vi "质控报警信息存储 (子VI).vi"   [LabVIEW 2016, in "质控单元.lvlib"]
uses:
  <vilib>/ptbypt/NI_PtbyPt.lvlib
types:
  T1 = cluster{"时间标识":timestamp, "设备":string, "日志信息":string, "流程参数":string}
  T2 = cluster{"时间标识":timestamp, "设备":string, "日志信息":string}
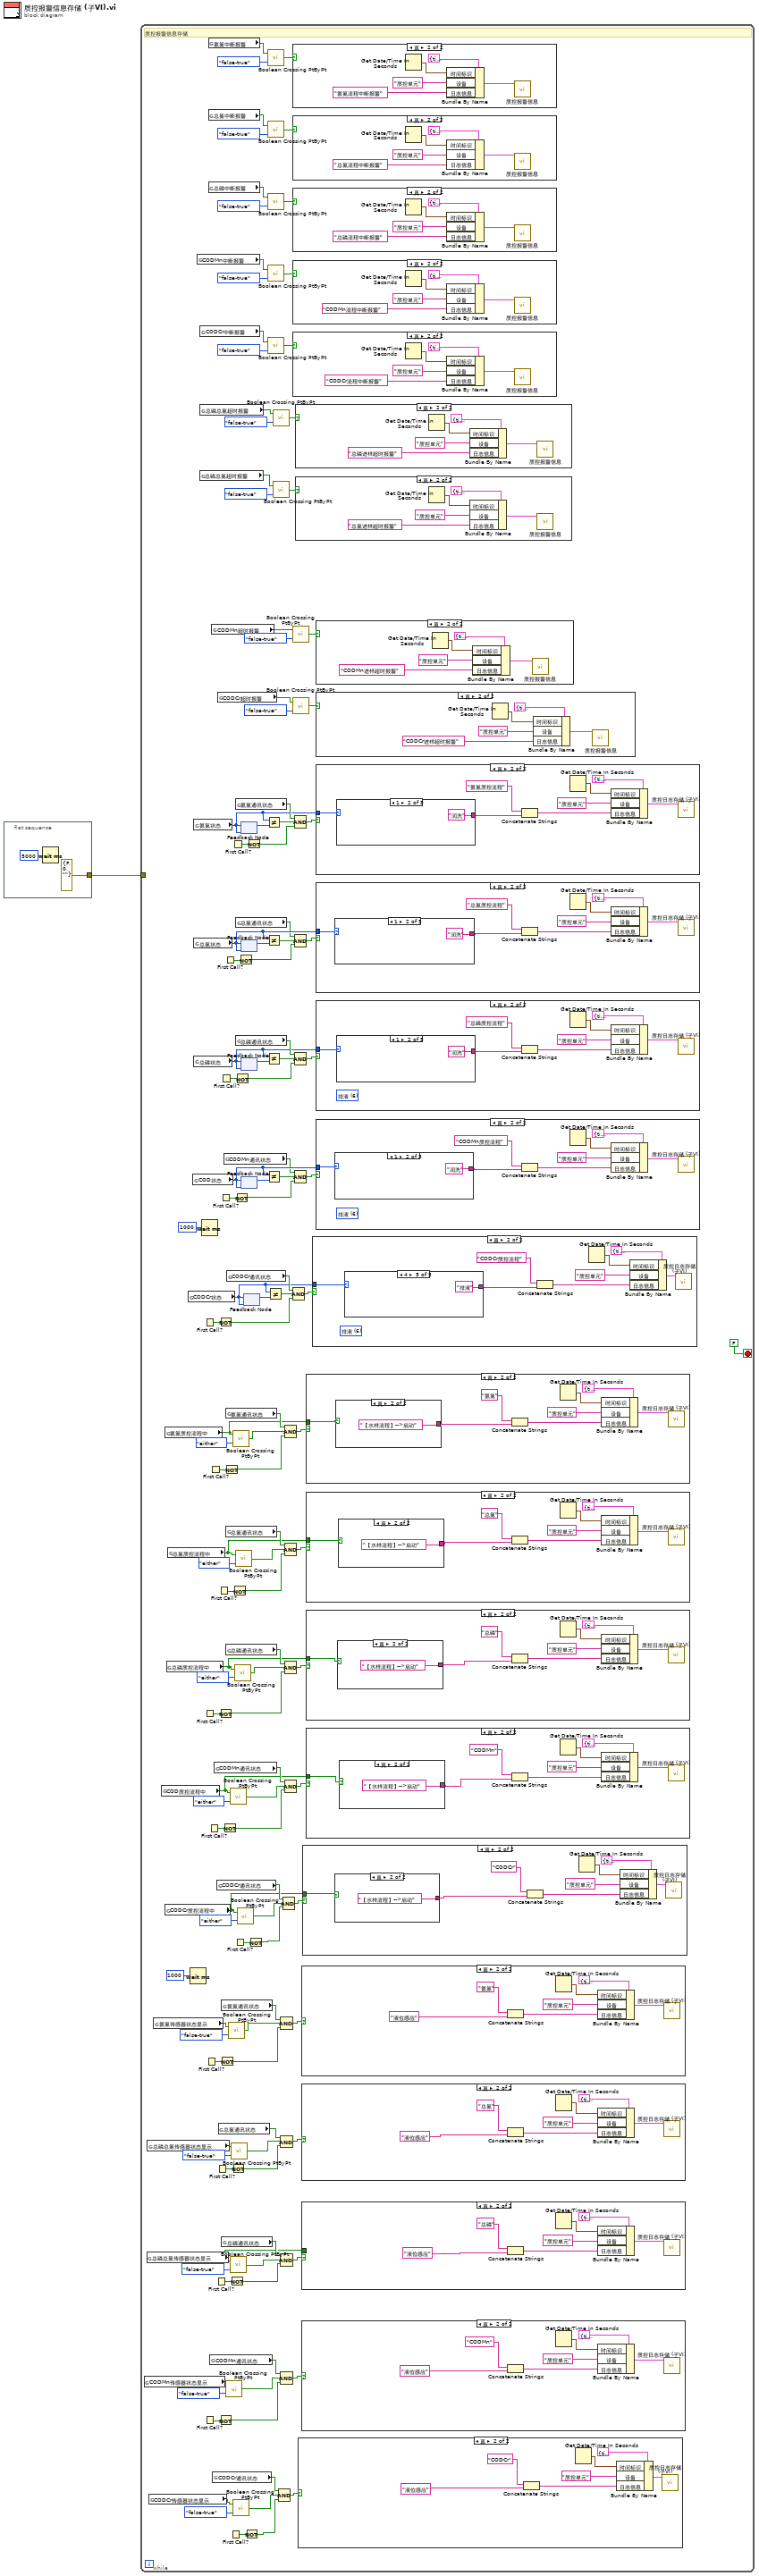
[diagram p0: block diagram]
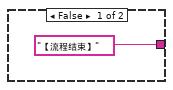
[diagram p8: hidden frame]
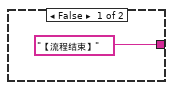
[diagram p10: hidden frame]
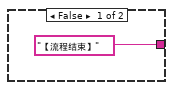
[diagram p12: hidden frame]
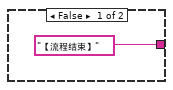
[diagram p14: hidden frame]
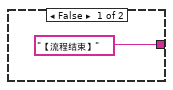
[diagram p16: hidden frame]
diagram:
  n1 = flat-sequence {
    tunnel: [errorcluster {"status"=FALSE, "code"=0, "source"=""} ("错误常量")] -> w1
    frame #0 {
      n2 = Wait (ms)(milliseconds to wait=u32 5000 ("等待时间（毫秒）")) -> ()  [unwired: 1 out]
    }
  }
  n3 = while {
    tunnel: w1 -> [_]
    stop <- FALSE stop-if-true
    # "质控报警信息存储"
    n4 = global read "质控中断报警全局.vi" "CODMn传感器状态显示"() -> (w5:bool)
    n5 = global read "质控中断报警全局.vi" "总磷总氮传感器状态显示"() -> (w6:bool)
    n6 = global read "质控中断报警全局.vi" "总磷总氮传感器状态显示"() -> (w7:bool)
    n7 = global read "质控中断报警全局.vi" "CODCr传感器状态显示"() -> (w4:bool)
    n8 = global read "质控中断报警全局.vi" "氨氮传感器状态显示"() -> (w8:bool)
    n9 = global read "质控测完标志全局 1.vi" "COD质控流程中"() -> (w42:bool)
    n10 = global read "质控测完标志全局 1.vi" "氨氮质控流程中"() -> (w51:bool)
    n11 = global read "质控测完标志全局 1.vi" "CODCr质控流程中"() -> (w40:bool)
    n12 = global read "质控测完标志全局 1.vi" "总磷质控流程中"() -> (w45:bool)
    n13 = global read "质控测完标志全局 1.vi" "总氮质控流程中"() -> (w48:bool)
    n14 = global read "加标回收状态全局变量.vi" "CODCr状态"() -> (w97:u16)
    n15 = Wait (ms)(milliseconds to wait=u32 1000 ("等待时间（毫秒）")) -> ()  [unwired: 1 out]
    n16 = global read "加标回收状态全局变量.vi" "COD状态"() -> (w106:u16)
    n17 = global read "加标回收状态全局变量.vi" "氨氮状态"() -> (w117:u16)
    n18 = global read "加标回收状态全局变量.vi" "总氮状态"() -> (w116:u16)
    n19 = global read "加标回收状态全局变量.vi" "总磷状态"() -> (w107:u16)
    n20 = global read "质控中断报警全局.vi" "CODMn中断报警"() -> (w130:bool)
    n21 = global read "质控中断报警全局.vi" "总磷总氮超时报警"() -> (w87:bool)
    n22 = global read "质控中断报警全局.vi" "CODCr中断报警"() -> (w128:bool)
    n23 = global read "质控中断报警全局.vi" "总磷总氮超时报警"() -> (w85:bool)
    n24 = Wait (ms)(milliseconds to wait=u32 1000 ("等待时间（毫秒）")) -> ()  [unwired: 1 out]
    n25 = First Call?() -> (First Call?: T/F=w65:bool)
    n26 = First Call?() -> (First Call?: T/F=w59:bool)
    n27 = First Call?() -> (First Call?: T/F=w22:bool)
    n28 = First Call?() -> (First Call?: T/F=w28:bool)
    n29 = First Call?() -> (First Call?: T/F=w57:bool)
    n30 = First Call?() -> (First Call?: T/F=w63:bool)
    n31 = global read "质控中断报警全局.vi" "氨氮中断报警"() -> (w136:bool)
    n32 = global read "质控中断报警全局.vi" "总氮中断报警"() -> (w134:bool)
    n33 = global read "质控中断报警全局.vi" "总磷中断报警"() -> (w132:bool)
    n34 = global read "质控内部交互全局.vi" "CODMn通讯状态"() -> (w31:bool)
    n35 = global read "质控中断报警全局.vi" "CODMn超时报警"() -> (w89:bool)
    n36 = global read "质控内部交互全局.vi" "CODCr通讯状态"() -> (w30:bool)
    n37 = First Call?() -> (First Call?: T/F=w24:bool)
    n38 = global read "质控内部交互全局.vi" "CODMn通讯状态"() -> (w76:bool)
    n39 = First Call?() -> (First Call?: T/F=w26:bool)
    n40 = First Call?() -> (First Call?: T/F=w61:bool)
    n41 = global read "质控内部交互全局.vi" "CODCr通讯状态"() -> (w75:bool)
    n42 = global read "质控中断报警全局.vi" "CODCr超时报警"() -> (w91:bool)
    n43 = Not(x=w65) -> (.not. x?=w64:bool)
    n44 = Not(x=w59) -> (.not. x?=w58:bool)
    n45 = Not(x=w22) -> (.not. x?=w21:bool)
    n46 = First Call?() -> (First Call?: T/F=w67:bool)
    n47 = global read "质控内部交互全局.vi" "总氮通讯状态"() -> (w35:bool)
    n48 = First Call?() -> (First Call?: T/F=w69:bool)
    n49 = Not(x=w28) -> (.not. x?=w27:bool)
    n50 = global read "质控内部交互全局.vi" "氨氮通讯状态"() -> (w38:bool)
    n51 = global read "质控内部交互全局.vi" "总磷通讯状态"() -> (w34:bool)
    n52 = Not(x=w57) -> (.not. x?=w56:bool)
    n53 = First Call?() -> (First Call?: T/F=w71:bool)
    n54 = Not(x=w63) -> (.not. x?=w62:bool)
    n55 = global read "质控内部交互全局.vi" "CODMn通讯状态"() -> (w103:bool)
    n56 = global read "质控内部交互全局.vi" "氨氮通讯状态"() -> (w83:bool)
    n57 = global read "质控内部交互全局.vi" "总氮通讯状态"() -> (w80:bool)
    n58 = global read "质控内部交互全局.vi" "总磷通讯状态"() -> (w79:bool)
    n59 = call <vilib>:"Boolean Crossing PtByPt.vi"("direction"=enum16{"either", "false-true", "true-false"}."false-true", "input"=w5) -> ("crossing"=w11:bool)  [unwired: 1 in]
    n60 = global read "质控内部交互全局.vi" "CODCr通讯状态"() -> (w100:bool)
    n61 = First Call?() -> (First Call?: T/F=w20:bool)
    n62 = call <vilib>:"Boolean Crossing PtByPt.vi"("direction"=enum16{"either", "false-true", "true-false"}."false-true", "input"=w8) -> ("crossing"=w17:bool)  [unwired: 1 in]
    n63 = Not(x=w24) -> (.not. x?=w23:bool)
    n64 = First Call?() -> (First Call?: T/F=w73:bool)
    n65 = call <vilib>:"Boolean Crossing PtByPt.vi"("direction"=enum16{"either", "false-true", "true-false"}."either", "input"=w42) -> ("crossing"=w43:bool)  [unwired: 1 in]
    n66 = Not(x=w26) -> (.not. x?=w25:bool)
    n67 = call <vilib>:"Boolean Crossing PtByPt.vi"("direction"=enum16{"either", "false-true", "true-false"}."false-true", "input"=w6) -> ("crossing"=w13:bool)  [unwired: 1 in]
    n68 = call <vilib>:"Boolean Crossing PtByPt.vi"("direction"=enum16{"either", "false-true", "true-false"}."false-true", "input"=w7) -> ("crossing"=w15:bool)  [unwired: 1 in]
    n69 = Not(x=w61) -> (.not. x?=w60:bool)
    n70 = First Call?() -> (First Call?: T/F=w55:bool)
    n71 = call <vilib>:"Boolean Crossing PtByPt.vi"("direction"=enum16{"either", "false-true", "true-false"}."either", "input"=w51) -> ("crossing"=w52:bool)  [unwired: 1 in]
    n72 = call <vilib>:"Boolean Crossing PtByPt.vi"("direction"=enum16{"either", "false-true", "true-false"}."false-true", "input"=w4) -> ("crossing"=w9:bool)  [unwired: 1 in]
    n73 = Not(x=w67) -> (.not. x?=w66:bool)
    n74 = Not(x=w69) -> (.not. x?=w68:bool)
    n75 = call <vilib>:"Boolean Crossing PtByPt.vi"("direction"=enum16{"either", "false-true", "true-false"}."either", "input"=w45) -> ("crossing"=w46:bool)  [unwired: 1 in]
    n76 = global read "质控内部交互全局.vi" "氨氮通讯状态"() -> (w120:bool)
    n77 = global read "质控内部交互全局.vi" "总氮通讯状态"() -> (w113:bool)
    n78 = global read "质控内部交互全局.vi" "总磷通讯状态"() -> (w110:bool)
    n79 = call <vilib>:"Boolean Crossing PtByPt.vi"("direction"=enum16{"either", "false-true", "true-false"}."either", "input"=w48) -> ("crossing"=w49:bool)  [unwired: 1 in]
    n80 = call <vilib>:"Boolean Crossing PtByPt.vi"("direction"=enum16{"either", "false-true", "true-false"}."either", "input"=w40) -> ("crossing"=w39:bool)  [unwired: 1 in]
    n81 = Not(x=w71) -> (.not. x?=w70:bool)
    n82 = feedback #1(w117) -> (w121:u16)
    n83 = feedback-in #1(w117) -> ()
    n84 = feedback #2(w116) -> (w112:u16)
    n85 = feedback-in #2(w116) -> ()
    n86 = feedback #3(w107) -> (w111:u16)
    n87 = feedback-in #3(w107) -> ()
    n88 = feedback #4(w106) -> (w102:u16)
    n89 = feedback-in #4(w106) -> ()
    n90 = feedback #5(w97) -> (w101:u16)
    n91 = feedback-in #5(w97) -> ()
    n92 = Not(x=w20) -> (.not. x?=w19:bool)
    n93 = Not(x=w73) -> (.not. x?=w72:bool)
    n94 = Not(x=w55) -> (.not. x?=w54:bool)
    n95 = Not Equal?(x=w117, y=w121) -> (x != y?=w119:bool)
    n96 = Not Equal?(x=w116, y=w112) -> (x != y?=w114:bool)
    n97 = Not Equal?(x=w107, y=w111) -> (x != y?=w109:bool)
    n98 = Not Equal?(x=w106, y=w102) -> (x != y?=w104:bool)
    n99 = call <vilib>:"Boolean Crossing PtByPt.vi"("direction"=enum16{"either", "false-true", "true-false"}."false-true", "input"=w136) -> ("crossing"=w126:bool)  [unwired: 1 in]
    n100 = call <vilib>:"Boolean Crossing PtByPt.vi"("direction"=enum16{"either", "false-true", "true-false"}."false-true", "input"=w134) -> ("crossing"=w125:bool)  [unwired: 1 in]
    n101 = call <vilib>:"Boolean Crossing PtByPt.vi"("direction"=enum16{"either", "false-true", "true-false"}."false-true", "input"=w132) -> ("crossing"=w124:bool)  [unwired: 1 in]
    n102 = call <vilib>:"Boolean Crossing PtByPt.vi"("direction"=enum16{"either", "false-true", "true-false"}."false-true", "input"=w130) -> ("crossing"=w123:bool)  [unwired: 1 in]
    n103 = call <vilib>:"Boolean Crossing PtByPt.vi"("direction"=enum16{"either", "false-true", "true-false"}."false-true", "input"=w128) -> ("crossing"=w122:bool)  [unwired: 1 in]
    n104 = Not Equal?(x=w97, y=w101) -> (x != y?=w99:bool)
    n105 = call <vilib>:"Boolean Crossing PtByPt.vi"("direction"=enum16{"either", "false-true", "true-false"}."false-true", "input"=w85) -> ("crossing"=w93:bool)  [unwired: 1 in]
    n106 = call <vilib>:"Boolean Crossing PtByPt.vi"("direction"=enum16{"either", "false-true", "true-false"}."false-true", "input"=w87) -> ("crossing"=w94:bool)  [unwired: 1 in]
    n107 = Compound Arithmetic op=AND ("复合运算")(w30, w9, w19) -> (w29:bool)
    n108 = Compound Arithmetic op=AND ("复合运算")(w38, w17, w27) -> (w37:bool)
    n109 = Compound Arithmetic op=AND ("复合运算")(w35, w15, w25) -> (w36:bool)
    n110 = Compound Arithmetic op=AND ("复合运算")(w34, w13, w23) -> (w33:bool)
    n111 = Compound Arithmetic op=AND ("复合运算")(w31, w11, w21) -> (w32:bool)
    n112 = Compound Arithmetic op=AND ("复合运算")(w75, w39, w54) -> (w74:bool)
    n113 = Compound Arithmetic op=AND ("复合运算")(w83, w52, w62) -> (w82:bool)
    n114 = Compound Arithmetic op=AND ("复合运算")(w80, w49, w60) -> (w81:bool)
    n115 = Compound Arithmetic op=AND ("复合运算")(w79, w46, w58) -> (w78:bool)
    n116 = Compound Arithmetic op=AND ("复合运算")(w76, w43, w56) -> (w77:bool)
    n117 = case shown="真" w126 {
      frame False {
      }
      frame True {
        n118 = Get Date/Time In Seconds() -> (seconds since 1Jan1904=w333:timestamp)
        n119 = Bundle By Name(cluster=T2 {"时间标识"=timestamp(0 s since 1904-01-01), "设备"="", "日志信息"=""} ("data in"), "时间标识"=w333, "设备"="质控单元", "日志信息"="氨氮流程中断报警") -> (w329:T2)
        n120 = call "质控报警信息.vi"("data in"=w329) -> ()  [unwired: 11 in]
      }
    }
    n121 = case shown="真" w125 {
      frame False {
      }
      frame True {
        n122 = Get Date/Time In Seconds() -> (seconds since 1Jan1904=w328:timestamp)
        n123 = Bundle By Name(cluster=T2 {"时间标识"=timestamp(0 s since 1904-01-01), "设备"="", "日志信息"=""} ("data in"), "时间标识"=w328, "设备"="质控单元", "日志信息"="总氮流程中断报警") -> (w324:T2)
        n124 = call "质控报警信息.vi"("data in"=w324) -> ()  [unwired: 11 in]
      }
    }
    n125 = case shown="真" w124 {
      frame False {
      }
      frame True {
        n126 = Get Date/Time In Seconds() -> (seconds since 1Jan1904=w323:timestamp)
        n127 = Bundle By Name(cluster=T2 {"时间标识"=timestamp(0 s since 1904-01-01), "设备"="", "日志信息"=""} ("data in"), "时间标识"=w323, "设备"="质控单元", "日志信息"="总磷流程中断报警") -> (w319:T2)
        n128 = call "质控报警信息.vi"("data in"=w319) -> ()  [unwired: 11 in]
      }
    }
    n129 = case shown="真" w123 {
      frame False {
      }
      frame True {
        n130 = Get Date/Time In Seconds() -> (seconds since 1Jan1904=w318:timestamp)
        n131 = Bundle By Name(cluster=T2 {"时间标识"=timestamp(0 s since 1904-01-01), "设备"="", "日志信息"=""} ("data in"), "时间标识"=w318, "设备"="质控单元", "日志信息"="CODMn流程中断报警") -> (w314:T2)
        n132 = call "质控报警信息.vi"("data in"=w314) -> ()  [unwired: 11 in]
      }
    }
    n133 = case shown="真" w122 {
      frame False {
      }
      frame True {
        n134 = Get Date/Time In Seconds() -> (seconds since 1Jan1904=w313:timestamp)
        n135 = Bundle By Name(cluster=T2 {"时间标识"=timestamp(0 s since 1904-01-01), "设备"="", "日志信息"=""} ("data in"), "时间标识"=w313, "设备"="质控单元", "日志信息"="CODCr流程中断报警") -> (w309:T2)
        n136 = call "质控报警信息.vi"("data in"=w309) -> ()  [unwired: 11 in]
      }
    }
    n137 = Compound Arithmetic op=AND ("复合运算")(w100, w99, w64) -> (w98:bool)
    n138 = call <vilib>:"Boolean Crossing PtByPt.vi"("direction"=enum16{"either", "false-true", "true-false"}."false-true", "input"=w89) -> ("crossing"=w95:bool)  [unwired: 1 in]
    n139 = call <vilib>:"Boolean Crossing PtByPt.vi"("direction"=enum16{"either", "false-true", "true-false"}."false-true", "input"=w91) -> ("crossing"=w96:bool)  [unwired: 1 in]
    n140 = Compound Arithmetic op=AND ("复合运算")(w120, w119, w72) -> (w118:bool)
    n141 = Compound Arithmetic op=AND ("复合运算")(w113, w114, w70) -> (w115:bool)
    n142 = Compound Arithmetic op=AND ("复合运算")(w110, w109, w68) -> (w108:bool)
    n143 = Compound Arithmetic op=AND ("复合运算")(w103, w104, w66) -> (w105:bool)
    n144 = case shown="真" w93 {
      frame False {
      }
      frame True {
        n145 = Get Date/Time In Seconds() -> (seconds since 1Jan1904=w243:timestamp)
        n146 = Bundle By Name(cluster=T2 {"时间标识"=timestamp(0 s since 1904-01-01), "设备"="", "日志信息"=""} ("data in"), "时间标识"=w243, "设备"="质控单元", "日志信息"="总磷进样超时报警") -> (w239:T2)
        n147 = call "质控报警信息.vi"("data in"=w239) -> ()  [unwired: 11 in]
      }
    }
    n148 = case shown="真" w94 {
      frame False {
      }
      frame True {
        n149 = Get Date/Time In Seconds() -> (seconds since 1Jan1904=w238:timestamp)
        n150 = Bundle By Name(cluster=T2 {"时间标识"=timestamp(0 s since 1904-01-01), "设备"="", "日志信息"=""} ("data in"), "时间标识"=w238, "设备"="质控单元", "日志信息"="总氮进样超时报警") -> (w234:T2)
        n151 = call "质控报警信息.vi"("data in"=w234) -> ()  [unwired: 11 in]
      }
    }
    n152 = case shown="真" w29 {
      frame False {
      }
      frame True {
        n153 = Concatenate Strings("CODCr" ("日志信息"), "液位感应" ("日志信息")) -> (w140:string)
        n154 = Get Date/Time In Seconds() -> (seconds since 1Jan1904=w143:timestamp)
        n155 = Bundle By Name(cluster=T1 {"时间标识"=timestamp(0 s since 1904-01-01), "设备"="", "日志信息"="", "流程参数"=""} ("data in"), "时间标识"=w143, "设备"="质控单元", "日志信息"=w140) -> (w144:T1)
        n156 = call "质控日志存储 (子VI).vi"("data in"=w144) -> ()  [unwired: 11 in]
      }
    }
    n157 = case shown="真" w37 {
      frame False {
      }
      frame True {
        n158 = Concatenate Strings("氨氮" ("日志信息"), "液位感应" ("日志信息")) -> (w168:string)
        n159 = Get Date/Time In Seconds() -> (seconds since 1Jan1904=w171:timestamp)
        n160 = Bundle By Name(cluster=T1 {"时间标识"=timestamp(0 s since 1904-01-01), "设备"="", "日志信息"="", "流程参数"=""} ("data in"), "时间标识"=w171, "设备"="质控单元", "日志信息"=w168) -> (w172:T1)
        n161 = call "质控日志存储 (子VI).vi"("data in"=w172) -> ()  [unwired: 11 in]
      }
    }
    n162 = case shown="真" w36 {
      frame False {
      }
      frame True {
        n163 = Concatenate Strings("总氮" ("日志信息"), "液位感应" ("日志信息")) -> (w161:string)
        n164 = Get Date/Time In Seconds() -> (seconds since 1Jan1904=w164:timestamp)
        n165 = Bundle By Name(cluster=T1 {"时间标识"=timestamp(0 s since 1904-01-01), "设备"="", "日志信息"="", "流程参数"=""} ("data in"), "时间标识"=w164, "设备"="质控单元", "日志信息"=w161) -> (w165:T1)
        n166 = call "质控日志存储 (子VI).vi"("data in"=w165) -> ()  [unwired: 11 in]
      }
    }
    n167 = case shown="真" w33 {
      tunnel: w6 -> [_ _]
      frame False {
      }
      frame True {
        n168 = Concatenate Strings("总磷" ("日志信息"), "液位感应" ("日志信息")) -> (w154:string)
        n169 = Get Date/Time In Seconds() -> (seconds since 1Jan1904=w157:timestamp)
        n170 = Bundle By Name(cluster=T1 {"时间标识"=timestamp(0 s since 1904-01-01), "设备"="", "日志信息"="", "流程参数"=""} ("data in"), "时间标识"=w157, "设备"="质控单元", "日志信息"=w154) -> (w158:T1)
        n171 = call "质控日志存储 (子VI).vi"("data in"=w158) -> ()  [unwired: 11 in]
      }
    }
    n172 = case shown="真" w32 {
      frame False {
      }
      frame True {
        n173 = Concatenate Strings("CODMn" ("日志信息"), "液位感应" ("日志信息")) -> (w147:string)
        n174 = Get Date/Time In Seconds() -> (seconds since 1Jan1904=w150:timestamp)
        n175 = Bundle By Name(cluster=T1 {"时间标识"=timestamp(0 s since 1904-01-01), "设备"="", "日志信息"="", "流程参数"=""} ("data in"), "时间标识"=w150, "设备"="质控单元", "日志信息"=w147) -> (w151:T1)
        n176 = call "质控日志存储 (子VI).vi"("data in"=w151) -> ()  [unwired: 11 in]
      }
    }
    n177 = case shown="真" w74 {
      tunnel: w40 -> [_ w175]
      frame False {
      }
      frame True {
        n178 = case shown="真" w175 {
          tunnel: ["【流程结束】" ("日志信息") "【水样流程】-->启动" ("日志信息")] -> w174
          frame False {
          }
          frame True {
          }
        }
        n179 = Concatenate Strings("CODCr" ("日志信息"), w174) -> (w176:string)
        n180 = Get Date/Time In Seconds() -> (seconds since 1Jan1904=w179:timestamp)
        n181 = Bundle By Name(cluster=T1 {"时间标识"=timestamp(0 s since 1904-01-01), "设备"="", "日志信息"="", "流程参数"=""} ("data in"), "时间标识"=w179, "设备"="质控单元", "日志信息"=w176) -> (w180:T1)
        n182 = call "质控日志存储 (子VI).vi"("data in"=w180) -> ()  [unwired: 11 in]
      }
    }
    n183 = case shown="真" w82 {
      tunnel: w51 -> [_ w215]
      frame False {
      }
      frame True {
        n184 = case shown="真" w215 {
          tunnel: ["【流程结束】" ("日志信息") "【水样流程】-->启动" ("日志信息")] -> w214
          frame False {
          }
          frame True {
          }
        }
        n185 = Concatenate Strings("氨氮" ("日志信息"), w214) -> (w216:string)
        n186 = Get Date/Time In Seconds() -> (seconds since 1Jan1904=w219:timestamp)
        n187 = Bundle By Name(cluster=T1 {"时间标识"=timestamp(0 s since 1904-01-01), "设备"="", "日志信息"="", "流程参数"=""} ("data in"), "时间标识"=w219, "设备"="质控单元", "日志信息"=w216) -> (w220:T1)
        n188 = call "质控日志存储 (子VI).vi"("data in"=w220) -> ()  [unwired: 11 in]
      }
    }
    n189 = case shown="真" w81 {
      tunnel: w48 -> [_ w205]
      frame False {
      }
      frame True {
        n190 = case shown="真" w205 {
          tunnel: ["【流程结束】" ("日志信息") "【水样流程】-->启动" ("日志信息")] -> w204
          frame False {
          }
          frame True {
          }
        }
        n191 = Concatenate Strings("总氮" ("日志信息"), w204) -> (w206:string)
        n192 = Get Date/Time In Seconds() -> (seconds since 1Jan1904=w209:timestamp)
        n193 = Bundle By Name(cluster=T1 {"时间标识"=timestamp(0 s since 1904-01-01), "设备"="", "日志信息"="", "流程参数"=""} ("data in"), "时间标识"=w209, "设备"="质控单元", "日志信息"=w206) -> (w210:T1)
        n194 = call "质控日志存储 (子VI).vi"("data in"=w210) -> ()  [unwired: 11 in]
      }
    }
    n195 = case shown="真" w78 {
      tunnel: w45 -> [_ w195]
      frame False {
      }
      frame True {
        n196 = case shown="真" w195 {
          tunnel: ["【流程结束】" ("日志信息") "【水样流程】-->启动" ("日志信息")] -> w194
          frame False {
          }
          frame True {
          }
        }
        n197 = Concatenate Strings("总磷" ("日志信息"), w194) -> (w196:string)
        n198 = Get Date/Time In Seconds() -> (seconds since 1Jan1904=w199:timestamp)
        n199 = Bundle By Name(cluster=T1 {"时间标识"=timestamp(0 s since 1904-01-01), "设备"="", "日志信息"="", "流程参数"=""} ("data in"), "时间标识"=w199, "设备"="质控单元", "日志信息"=w196) -> (w200:T1)
        n200 = call "质控日志存储 (子VI).vi"("data in"=w200) -> ()  [unwired: 11 in]
      }
    }
    n201 = case shown="真" w77 {
      tunnel: w42 -> [_ w185]
      frame False {
      }
      frame True {
        n202 = case shown="真" w185 {
          tunnel: ["【流程结束】" ("日志信息") "【水样流程】-->启动" ("日志信息")] -> w184
          frame False {
          }
          frame True {
          }
        }
        n203 = Concatenate Strings("CODMn" ("日志信息"), w184) -> (w186:string)
        n204 = Get Date/Time In Seconds() -> (seconds since 1Jan1904=w189:timestamp)
        n205 = Bundle By Name(cluster=T1 {"时间标识"=timestamp(0 s since 1904-01-01), "设备"="", "日志信息"="", "流程参数"=""} ("data in"), "时间标识"=w189, "设备"="质控单元", "日志信息"=w186) -> (w190:T1)
        n206 = call "质控日志存储 (子VI).vi"("data in"=w190) -> ()  [unwired: 11 in]
      }
    }
    n207 = case shown="真" w98 {
      tunnel: w97 -> [_ w245]
      frame False {
      }
      frame True {
        (unwired) u16 6 items=["待机", "润洗", "进样", "进样完成", "柱塞泵加标", "等待取液", "排液"] ("氨氮状态")
        n208 = case shown="4" w245 {
          tunnel: ["结束" ("日志信息") "润洗" ("日志信息") "进样" ("日志信息") "等待取样" ("日志信息") "排液" ("日志信息")] -> w244
          frame 0, Default {
          }
          frame 1 {
          }
          frame 2 {
          }
          frame 3 {
          }
          frame 4 {
          }
        }
        n209 = Concatenate Strings("CODCr质控流程" ("日志信息"), w244) -> (w246:string)
        n210 = Get Date/Time In Seconds() -> (seconds since 1Jan1904=w249:timestamp)
        n211 = Bundle By Name(cluster=T1 {"时间标识"=timestamp(0 s since 1904-01-01), "设备"="", "日志信息"="", "流程参数"=""} ("data in"), "时间标识"=w249, "设备"="质控单元", "日志信息"=w246) -> (w250:T1)
        n212 = call "质控日志存储 (子VI).vi"("data in"=w250) -> ()  [unwired: 11 in]
      }
    }
    n213 = case shown="真" w95 {
      frame False {
      }
      frame True {
        n214 = Get Date/Time In Seconds() -> (seconds since 1Jan1904=w233:timestamp)
        n215 = Bundle By Name(cluster=T2 {"时间标识"=timestamp(0 s since 1904-01-01), "设备"="", "日志信息"=""} ("data in"), "时间标识"=w233, "设备"="质控单元", "日志信息"="CODMn进样超时报警") -> (w229:T2)
        n216 = call "质控报警信息.vi"("data in"=w229) -> ()  [unwired: 11 in]
      }
    }
    n217 = case shown="真" w96 {
      frame False {
      }
      frame True {
        n218 = Get Date/Time In Seconds() -> (seconds since 1Jan1904=w228:timestamp)
        n219 = Bundle By Name(cluster=T2 {"时间标识"=timestamp(0 s since 1904-01-01), "设备"="", "日志信息"=""} ("data in"), "时间标识"=w228, "设备"="质控单元", "日志信息"="CODCr进样超时报警") -> (w224:T2)
        n220 = call "质控报警信息.vi"("data in"=w224) -> ()  [unwired: 11 in]
      }
    }
    n221 = case shown="真" w118 {
      tunnel: w117 -> [_ w299]
      frame False {
      }
      frame True {
        n222 = case shown="1" w299 {
          tunnel: ["结束" ("日志信息") "润洗" ("日志信息") "进样" ("日志信息") "等待取样" ("日志信息") "排液" ("日志信息")] -> w297
          frame 0, Default {
          }
          frame 1 {
          }
          frame 2 {
          }
          frame 3 {
          }
          frame 4 {
          }
        }
        n223 = Concatenate Strings("氨氮质控流程" ("日志信息"), w297) -> (w296:string)
        n224 = Get Date/Time In Seconds() -> (seconds since 1Jan1904=w301:timestamp)
        n225 = Bundle By Name(cluster=T1 {"时间标识"=timestamp(0 s since 1904-01-01), "设备"="", "日志信息"="", "流程参数"=""} ("data in"), "时间标识"=w301, "设备"="质控单元", "日志信息"=w296) -> (w302:T1)
        n226 = call "质控日志存储 (子VI).vi"("data in"=w302) -> ()  [unwired: 11 in]
      }
    }
    n227 = case shown="真" w115 {
      tunnel: w116 -> [_ w284]
      frame False {
      }
      frame True {
        n228 = case shown="1" w284 {
          tunnel: ["结束" ("日志信息") "润洗" ("日志信息") "进样" ("日志信息") "等待取样" ("日志信息") "排液" ("日志信息")] -> w283
          frame 0, Default {
          }
          frame 1 {
          }
          frame 2 {
          }
          frame 3 {
          }
          frame 4 {
          }
        }
        n229 = Concatenate Strings("总氮质控流程" ("日志信息"), w283) -> (w285:string)
        n230 = Get Date/Time In Seconds() -> (seconds since 1Jan1904=w288:timestamp)
        n231 = Bundle By Name(cluster=T1 {"时间标识"=timestamp(0 s since 1904-01-01), "设备"="", "日志信息"="", "流程参数"=""} ("data in"), "时间标识"=w288, "设备"="质控单元", "日志信息"=w285) -> (w289:T1)
        n232 = call "质控日志存储 (子VI).vi"("data in"=w289) -> ()  [unwired: 11 in]
      }
    }
    n233 = case shown="真" w108 {
      tunnel: w107 -> [_ w271]
      frame False {
      }
      frame True {
        (unwired) u16 6 items=["待机", "润洗", "进样", "进样完成", "柱塞泵加标", "等待取液", "排液"] ("氨氮状态")
        n234 = case shown="1" w271 {
          tunnel: ["结束" ("日志信息") "润洗" ("日志信息") "进样" ("日志信息") "等待取样" ("日志信息") "排液" ("日志信息")] -> w270
          frame 0, Default {
          }
          frame 1 {
          }
          frame 2 {
          }
          frame 3 {
          }
          frame 4 {
          }
        }
        n235 = Concatenate Strings("总磷质控流程" ("日志信息"), w270) -> (w272:string)
        n236 = Get Date/Time In Seconds() -> (seconds since 1Jan1904=w275:timestamp)
        n237 = Bundle By Name(cluster=T1 {"时间标识"=timestamp(0 s since 1904-01-01), "设备"="", "日志信息"="", "流程参数"=""} ("data in"), "时间标识"=w275, "设备"="质控单元", "日志信息"=w272) -> (w276:T1)
        n238 = call "质控日志存储 (子VI).vi"("data in"=w276) -> ()  [unwired: 11 in]
      }
    }
    n239 = case shown="真" w105 {
      tunnel: w106 -> [_ w258]
      frame False {
      }
      frame True {
        (unwired) u16 6 items=["待机", "润洗", "进样", "进样完成", "柱塞泵加标", "等待取液", "排液"] ("氨氮状态")
        n240 = case shown="1" w258 {
          tunnel: ["结束" ("日志信息") "润洗" ("日志信息") "进样" ("日志信息") "等待取样" ("日志信息") "排液" ("日志信息")] -> w257
          frame 0, Default {
          }
          frame 1 {
          }
          frame 2 {
          }
          frame 3 {
          }
          frame 4 {
          }
        }
        n241 = Concatenate Strings("CODMn质控流程" ("日志信息"), w257) -> (w259:string)
        n242 = Get Date/Time In Seconds() -> (seconds since 1Jan1904=w262:timestamp)
        n243 = Bundle By Name(cluster=T1 {"时间标识"=timestamp(0 s since 1904-01-01), "设备"="", "日志信息"="", "流程参数"=""} ("data in"), "时间标识"=w262, "设备"="质控单元", "日志信息"=w259) -> (w263:T1)
        n244 = call "质控日志存储 (子VI).vi"("data in"=w263) -> ()  [unwired: 11 in]
      }
    }
  }
